vi "OPCReadLab.vi"() -> ()   [LabVIEW 2021]
panel:
  out "Query":string caption="Result"
  out "OPC Read":dbl
  in  "stop":bool
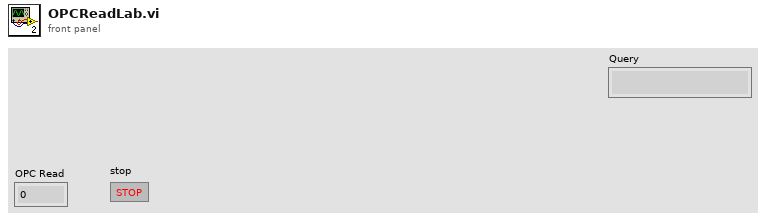
[diagram p1: front panel]
types:
  T1 = enum16{"Read", "Write", "ReadWrite", "BufferedRead", "BufferedReadWrite"}
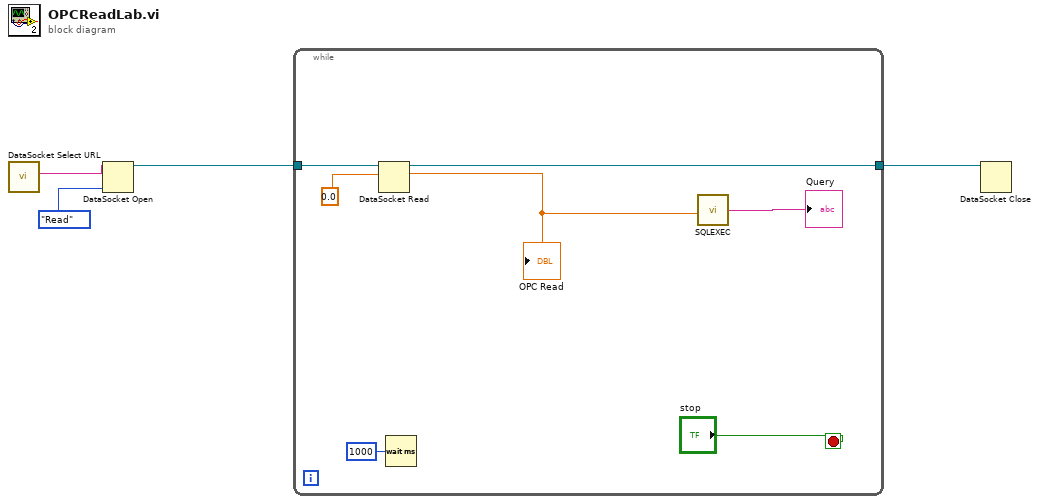
[diagram p0: block diagram]
diagram:
  n1 = call <vilib>:"DataSocket Select URL.vi"() -> ("URL"=w4:string)  [unwired: 9 in, 2 out]
  n2 = DataSocket Open(10:T1."Read" ("mode"), 11:w4) -> (3:w2:refnum<k13>)  [unwired: 2 in, 1 out]
  n3 = while {
    tunnel: w2 -> [w11]
    tunnel: [w8] -> w1
    stop <- "stop" stop-if-true
    n4 = DataSocket Read(10:0.0, 11:w11) -> (2:w6:dbl, 3:w8:refnum<k13>)  [unwired: 3 in, 5 out]
    "OPC Read" <- w6
    n5 = Wait (ms)(milliseconds to wait=u32 1000) -> ()  [unwired: 1 out]
    n6 = call "SQLEXEC.vi"("value"=w6) -> ("Query"=→"Query":string)  [unwired: 1 in]
  }
  n7 = DataSocket Close(11:w1) -> ()  [unwired: 2 in, 2 out]
